vi "Rollers Controller.vi"(8 "error in":errorcluster) -> ()   [LabVIEW 2018]
doc: "This VI executes continuously carrying out the current operation and responding to updates or new operations. It will often contain the timing or control code that is difficult to place directly in TeleOp. This VI generally opens all sensors and motors and isolates the rest of the robot code from knowing how the operations are carried out."
uses:
  <vilib>/Rock Robotics/WPI/Framework/Completion Status.ctl
  Rollers Setpoints.ctl
  Rollers Operations.ctl
  <vilib>/Rock Robotics/WPI/SafetyOutput/WPI_SafetyOutputConfigMenu.ctl
  <vilib>/Rock Robotics/WPI/MotorControl/WPI_MotorControlDeviceRef.ctl
  <vilib>/Rock Robotics/WPI/MotorControl/WPI_MotorControlType.ctl
  <vilib>/Rock Robotics/SystemInterfaces/DIO/FPGA_DIOPWMChannel.ctl
  <vilib>/Rock Robotics/WPI/PWM/WPI_PWMDeadband.ctl
  <vilib>/Rock Robotics/SystemInterfaces/DIO/FPGA_DIOChannel.ctl
panel:
  in  "Shoot Speed":dbl=0.3
  in  "Intake Speed":dbl=-0.6
  in  "Interactive Values":T1
  out "Current\nCmd":string
  in  "Buttons":cluster{"Execute Cmd":bool, "Abort Cmd":bool}
  out "Command Timing":cluster{"Start Time (ms)":u32, "Iterations":i32}
  out "Status":T3
  # "Interactive Command: You may fill in the settings for a command\nand schedule it with the Execute button. You can observe and abort\nany command while fine tuning the code for the controller."
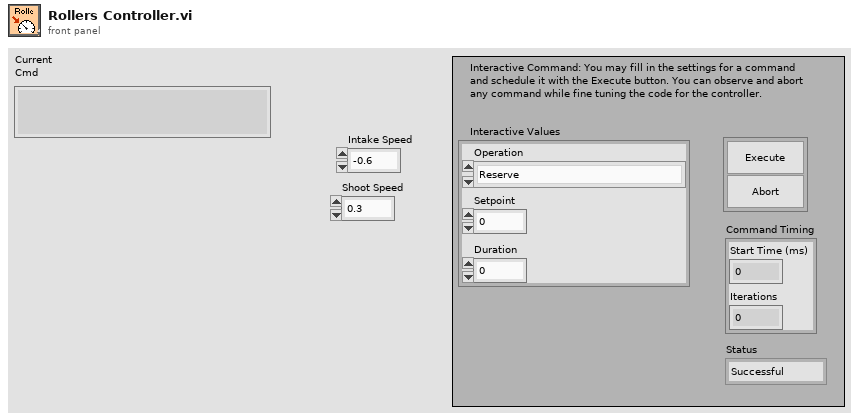
[diagram p1: front panel]
types:
  T1 = typedef "Rollers Setpoints.ctl" = cluster{"Operation":T2, "Setpoint":dbl, "Duration":dbl}
  T2 = typedef "Rollers Operations.ctl" = enum16{"Reserve", "Read Current", "Immediate", "In", "Out", "Off", "Set Speed"}
  T3 = typedef "Completion Status.ctl" = enum16{"Successful", "Aborted", "Incomplete"}
  T4 = typedef "WPI_MotorControlDeviceRef.ctl" = cluster{"DeviceStatus":errorcluster, "Type":T5, "PWM":cluster{"PWM Channel":T6, "DeadBand":T7}, "CAN":cluster{"Device Number":u8, "SetOutput VI Ref":variant, "GetOutput VI Ref":variant, "Enable VI Ref":variant, "Disable VI Ref":variant, "Data":variant}, "Invert":bool, "DIO PWM":cluster{"PWM \"Enable\" Channel":T6, "DIOChannel":T8, "PWM Rate":dbl}}
  T5 = typedef "WPI_MotorControlType.ctl" = enum16{"PWM", "CAN", "DIO PWM"}
  T6 = typedef "FPGA_DIOPWMChannel.ctl" = enum8{"PWM 0", "PWM 1", "PWM 2", "PWM 3", "PWM 4", "PWM 5", "PWM 6", "PWM 7", "PWM 8", "PWM 9", "PWM MXP 0", "PWM MXP 1", "PWM MXP 2", "PWM MXP 3", "PWM MXP 4", "PWM MXP 5", "PWM MXP 6", "PWM MXP 7", "PWM MXP 8", "PWM MXP 9", "Invalid"}
  T7 = typedef "WPI_PWMDeadband.ctl" = cluster{"Name":string, "maxPositivePwm":i32, "minPositivePwm":i32, "centerPwm":i32, "maxNegativePwm":i32, "minNegativePwm":i32, "angularRange":u16}
  T8 = typedef "FPGA_DIOChannel.ctl" = enum8{"DIO 0", "DIO 1", "DIO 2", "DIO 3", "DIO 4", "DIO 5", "DIO 6", "DIO 7", "DIO 8", "DIO 9", "DIO MXP 0", "DIO MXP 1", "DIO MXP 2", "DIO MXP 3", "DIO MXP 4", "DIO MXP 5", "DIO MXP 6", "DIO MXP 7", "DIO MXP 8", "DIO MXP 9", "DIO MXP 10", "DIO MXP 11", "DIO MXP 12", "DIO MXP 13", "DIO MXP 14", "DIO MXP 15", "SPI Port CS1", "SPI Port CS2", "SPI Port CS3", "SPI Port MISO", "SPI Port MOSI", "Invalid"}
  T9 = typedef "WPI_SafetyOutputConfigMenu.ctl" = enum16{"Enable", "Disable"}
  T10 = typedef "Command Status Info.ctl" = cluster{"Name":string, "Status":T3, "notifier out":T11}
  T11 = typedef "Completion Notifier.ctl" = refnum<notifier>
  T12 = cluster{"Current Command":T1, "Command Timing":cluster{"Start Time (ms)":u32, "Iterations":i32}, "Command Arguments":cluster{"Command Info":T10, "Description":string, "Default Command":T1, "queue out":refnum<queue>, "Subsystem Name":string}}
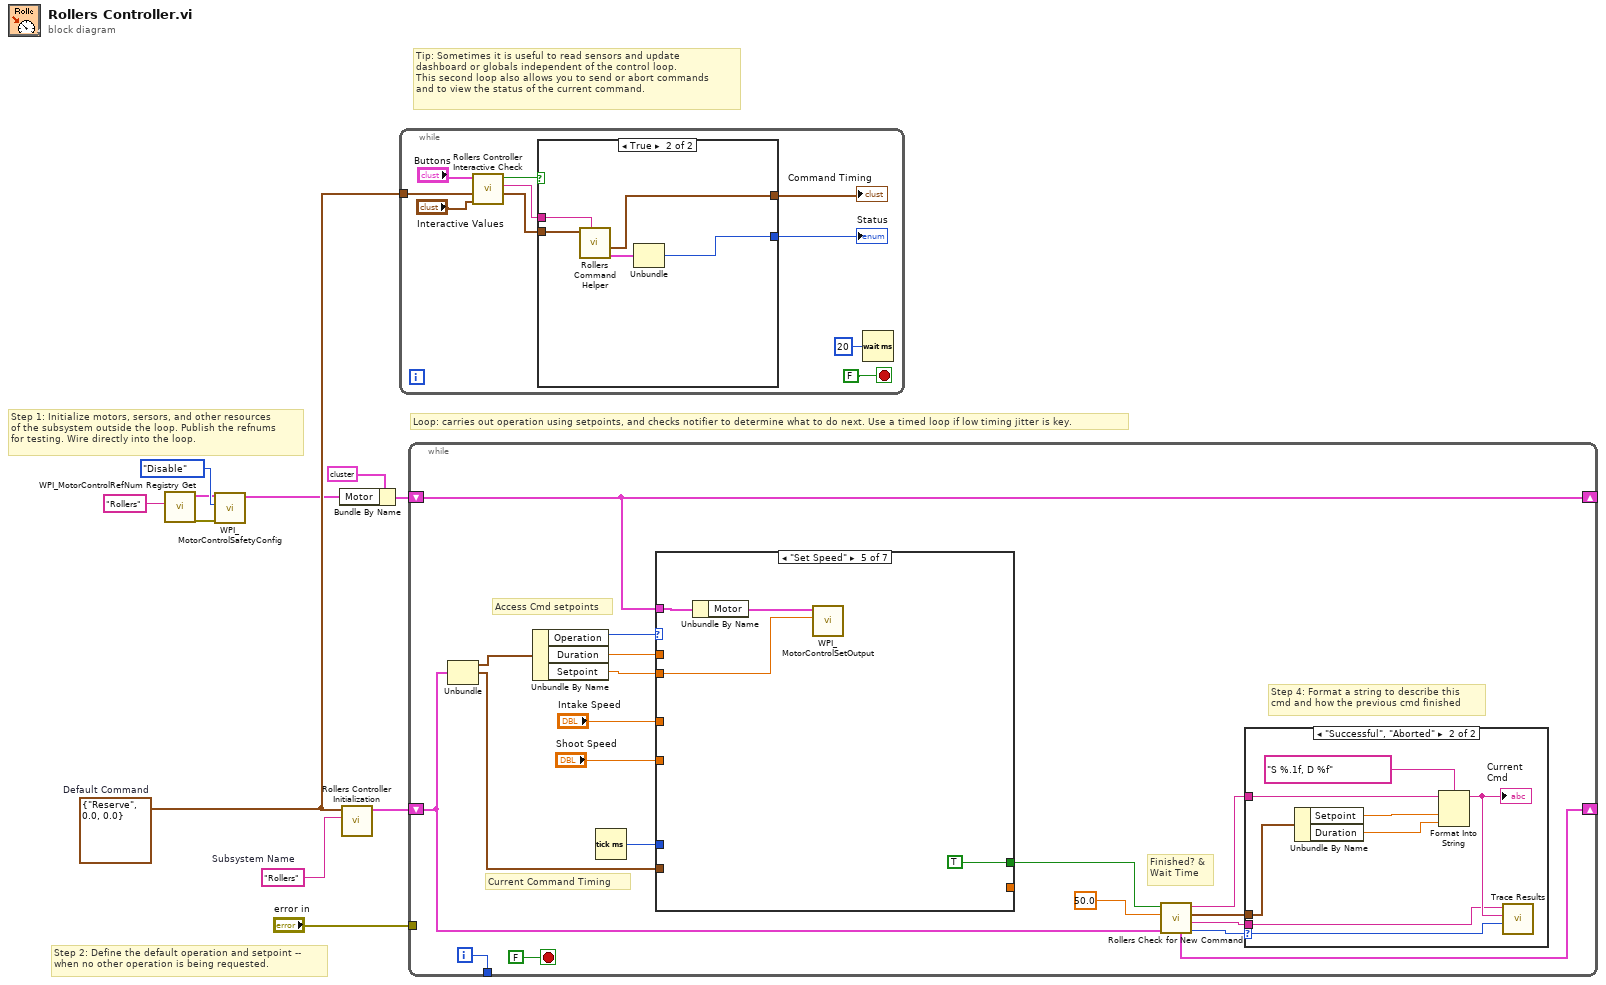
[diagram p0: block diagram]
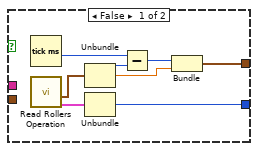
[diagram p2: hidden frame]
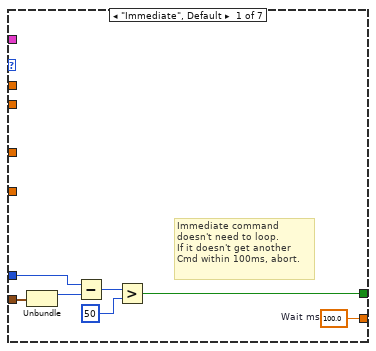
[diagram p4: hidden frame]
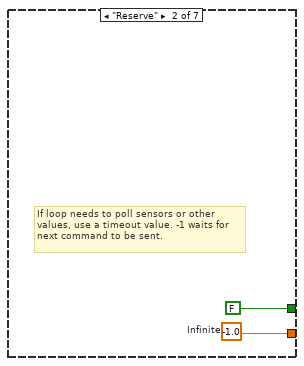
[diagram p5: hidden frame]
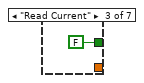
[diagram p6: hidden frame]
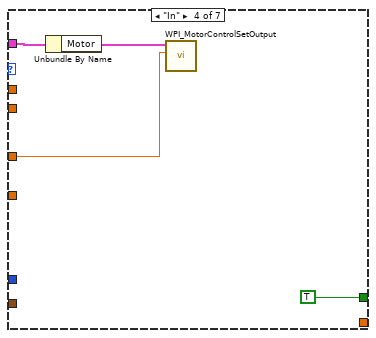
[diagram p7: hidden frame]
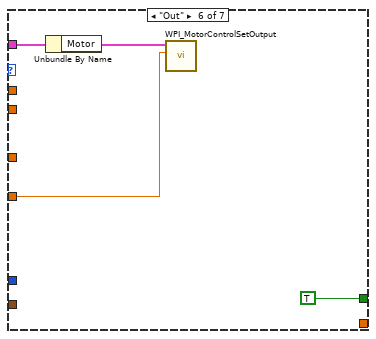
[diagram p8: hidden frame]
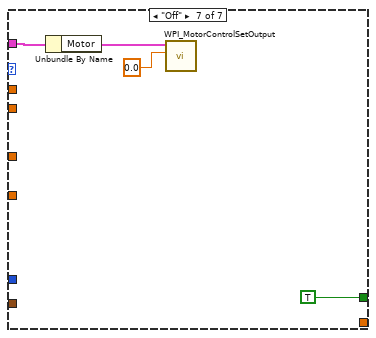
[diagram p9: hidden frame]
diagram:
  w8 = T1 {"Operation"=enum."Reserve", "Setpoint"=0.0, "Duration"=0.0}  # Default Command
  w9 = "Rollers"  # Subsystem Name
  # "Tip: Sometimes it is useful to read sensors and update\ndashboard or globals independent of the control loop.\nThis second loop also allows you to send or abort commands\nand to view the status of the current command."
  # "Step 2: Define the default operation and setpoint --\nwhen no other operation is being requested."
  # "Step 1: Initialize motors, sersors, and other resources\nof the subsystem outside the loop. Publish the refnums\nfor testing. Wire directly into the loop."
  # "Loop: carries out operation using setpoints, and checks notifier to determine what to do next. Use a timed loop if low timing jitter is key."
  n1 = call <vilib>:"WPI_MotorControlRefNum Registry Get.vi"("refnum name"="Rollers") -> ("error out"=w4:errorcluster, "MotorControlDevRef"=w5:T4)  [unwired: 9 in]
  n2 = call <vilib>:"WPI_MotorControlSafetyConfig.vi"("error in (no error)"=w4, "mode"=WPI_SafetyOutputConfigMenu."Disable", "MotorControlDevRef"=w5) -> ("MotorControlDevRef"=w2:T4)  [unwired: 7 in, 1 out]
  n3 = Bundle By Name(cluster=cluster{"Motor":T4, "Has Cargo?":bool} {"Motor"={"DeviceStatus"={"status"=FALSE, "code"=0, "source"=""}, "Type"=enum."PWM", "PWM"={"PWM Channel"=enum."Invalid", "DeadBand"={"Name"="", "maxPositivePwm"=0, "minPositivePwm"=0, "centerPwm"=0, "maxNegativePwm"=0, "minNegativePwm"=0, "angularRange"=0}}, "CAN"={"Device Number"=0, "SetOutput VI Ref"=variant(enum8{"Percent VBus", "Current", "Speed", "Position", "Voltage"} enum."Percent VBus"), "GetOutput VI Ref"=variant(refnum<k1> refnum), "Enable VI Ref"=variant(dbl 12.0), "Disable VI Ref"=variant(enum8{"Percent VBus", "Speed", "Position", "Slave", "Unchanged / Invalid", "Voltage Compensation", "Current", "Motion Profile"} enum."Percent VBus"), "Data"=variant}, "Invert"=FALSE, "DIO PWM"={"PWM \"Enable\" Channel"=enum."Invalid", "DIOChannel"=enum."Invalid", "PWM Rate"=0.0}}, "Has Cargo?"=FALSE}, "Motor"=w2) -> (w1:cluster{"Motor":T4, "Has Cargo?":bool})
  n4 = call "Rollers Controller Initialization.vi"("Subsystem Name"=w9, "Default Command"=w8) -> ("Current Command"=w10:T12)  [unwired: 9 in]
  n5 = while {
    tunnel: w8 -> [w18]
    stop <- FALSE stop-if-true
    n6 = call "Rollers Controller Interactive Check.vi"("Interactive Command in"="Interactive Values", "Default Command"=w18, "Buttons"="Buttons") -> ("Interactive Command out"=w15:T1, "Trace String"=w16:string, "Schedule"=w17:bool)  [unwired: 6 in]
    n7 = case shown="True" w17 {
      tunnel: [w29 w34] -> w14
      tunnel: w15 -> [_ w32]
      tunnel: [w25 w30] -> w13
      tunnel: w16 -> [_ w33]
      frame False {
        n8 = Tick Count (ms)() -> (millisecond timer value=w24:u32)
        n9 = call "Read Rollers Operation.vi"() -> ("Command Info"=w22:T10, "SubSystem Data"=w23:T1)  [unwired: 9 in, 1 out]
        n10 = Unbundle(w23) -> ("Operation"=w28:T2, "Setpoint"=w26:dbl)  [unwired: 1 out]
        n11 = Unbundle(w22) -> ("Status"=w29:T3)  [unwired: 2 out]
        n12 = Subtract(x=w24, y=w28) -> (x-y=w27:u32)
        n13 = Bundle(w27, "Setpoint"=w26) -> (w25:cluster{u32, "Setpoint":dbl})  [unwired: 1 in]
      }
      frame True {
        n14 = call "Rollers Command Helper.vi"("Description"=w33, "SubSystem Data"=w32) -> ("Command Info Out"=w31:T10, "Command Timing"=w30:cluster{"Start Time (ms)":u32, "Iterations":i32})  [unwired: 7 in, 1 out]
        n15 = Unbundle(w31) -> ("Status"=w34:T3)  [unwired: 2 out]
      }
    }
    "Status" <- w14
    "Command Timing" <- w13
    n16 = Wait (ms)(milliseconds to wait=u32 20) -> ()  [unwired: 1 out]
  }
  n17 = while {
    shift-right: [w45] -> _
    shift-left: w10 -> [w39]
    tunnel: [w52] -> _
    tunnel: "error in" -> [_]
    shift-right: [w37] -> _
    shift-left: w1 -> [w37]
    i -> [w52]
    stop <- FALSE stop-if-true
    # "Step 4: Format a string to describe this\ncmd and how the previous cmd finished"
    # "Current Command Timing"
    # "Access Cmd setpoints"
    # "Finished? &\nWait Time"
    n18 = Unbundle(w39) -> ("Current Command"=w51:T1, "Command Timing"=w47:cluster{"Start Time (ms)":u32, "Iterations":i32})  [unwired: 1 out]
    n19 = Unbundle By Name(w51) -> ("Operation"=w50:T2, "Duration"=w49:dbl, "Setpoint"=w46:dbl)
    n20 = Tick Count (ms)() -> (millisecond timer value=w48:u32)
    n21 = case shown="\"Set Speed\"" w50 {
      tunnel: [w68 w70 _ _ _ _ _] -> _
      tunnel: [w62 FALSE ("ignore previous (F)") FALSE ("ignore previous (F)") TRUE ("ignore previous (F)") TRUE ("ignore previous (F)") TRUE ("ignore previous (F)") TRUE ("ignore previous (F)")] -> w44
      tunnel: w47 -> [w64 _ _ _ _ _ _]
      tunnel: w49 -> [_ _ _ _ _ _ _]
      tunnel: w48 -> [w63 _ _ _ _ _ _]
      tunnel: w46 -> [_ _ _ _ w76 _ _]
      tunnel: w37 -> [_ _ _ w74 w78 w82 w86]
      tunnel: "Intake Speed" -> [_ _ _ w72 _ _ _]
      tunnel: "Shoot Speed" -> [_ _ _ _ _ w80 _]
      frame "Immediate", Default {
        w68 = 100.0  # Wait ms
        # "Immediate command\ndoesn't need to loop.\nIf it doesn't get another\nCmd within 100ms, abort."
        n22 = Unbundle(w64) -> ("Start Time (ms)"=w67:u32)  [unwired: 1 out]
        n23 = Subtract(x=w63, y=w67) -> (x-y=w66:u32)
        n24 = Greater?(x=w66, y=u8 50 ("Left Motor")) -> (0:w62:bool)
      }
      frame "Reserve" {
        w70 = -1.0  # Infinite
        # "If loop needs to poll sensors or other\nvalues, use a timeout value. -1 waits for\nnext command to be sent."
      }
      frame "Read Current" {
      }
      frame "In" {
        n25 = Unbundle By Name(w74) -> ("Motor"=w73:T4)
        n26 = call <vilib>:"WPI_MotorControlSetOutput.vi"("Output"=w72, "MotorControlDevRef"=w73) -> ()  [unwired: 7 in, 3 out]
      }
      frame "Set Speed" {
        n27 = Unbundle By Name(w78) -> ("Motor"=w77:T4)
        n28 = call <vilib>:"WPI_MotorControlSetOutput.vi"("Output"=w76, "MotorControlDevRef"=w77) -> ()  [unwired: 7 in, 3 out]
      }
      frame "Out" {
        n29 = Unbundle By Name(w82) -> ("Motor"=w81:T4)
        n30 = call <vilib>:"WPI_MotorControlSetOutput.vi"("Output"=w80, "MotorControlDevRef"=w81) -> ()  [unwired: 7 in, 3 out]
      }
      frame "Off" {
        n31 = Unbundle By Name(w86) -> ("Motor"=w85:T4)
        n32 = call <vilib>:"WPI_MotorControlSetOutput.vi"("Output"=0.0, "MotorControlDevRef"=w85) -> ()  [unwired: 7 in, 3 out]
      }
    }
    n33 = call "Rollers Check for New Command.vi"("Current Command"=w39, "Wait time (ms)"=50.0, "Finished?"=w44) -> ("Completion"=w40:T3, "Subsystem Name"=w41:string, "Current Command"=w42:T1, "Initial Trace String"=w43:string, "NextCommand"=w45:T12)  [unwired: 4 in]
    n34 = case shown="\"Successful\", \"Aborted\"" w40 {
      selector: w40 -> [_ w61]
      tunnel: w43 -> [_ w57]
      tunnel: w42 -> [_ w58]
      tunnel: w41 -> [_ w54]
      frame "Incomplete", Default {
        # "Continuing current command"
      }
      frame "Successful", "Aborted" {
        # "Report and setup for next command"
        n35 = Unbundle By Name(w58) -> ("Setpoint"=w60:dbl, "Duration"=w55:dbl)
        n36 = Format Into String(format string="S %.1f, D %f", initial string=w57, w60, w55) -> (resulting string=w56:string)  [unwired: 1 in, 1 out]
        "Current\nCmd" <- w56
        n37 = call <vilib>:"Trace Results.vi"("Status of previous command"=w61, "Description"=w56, "Subsystem"=w54) -> ()  [unwired: 9 in]
      }
    }
  }
